vi "Check Upgrade.vi"(8 "error in (no error)":errorcluster, 11 "WebSocket Client in":refnum<class "WebSocket Client.lvclass">) -> (0 "error out":errorcluster, 1 "Is WS Upgrade":bool, 2 "Response":refnum<class "WebSocketUpgradeResponse.lvclass">, 3 "WebSocket Client out":refnum<class "WebSocket Client.lvclass">)   [LabVIEW 2020, in "HTTP Server.lvlib" / "WebSocket Client.lvclass"]
uses:
  WebSocket Client.lvclass
  WebSocket Client.lvclass/WebSocket Client.ctl
  lv-http-util/HTTP Utils/Request/Request.lvclass
  lv-http-util/HTTP Utils/Method.ctl
  lv-http-util/HTTP Utils/HTTP Utils.lvlib
  WebSocketUpgradeResponse/WebSocketUpgradeResponse.lvclass
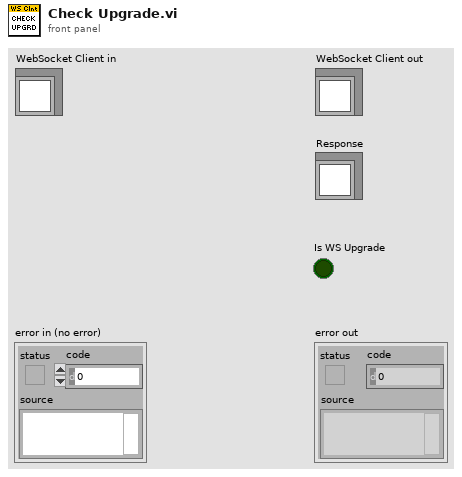
[diagram p1: front panel]
types:
  T1 = typedef "HTTP Utils.lvlib/Method.ctl" = enum16{"GET", "HEAD", "POST", "PUT", "DELETE", "CONNECT", "OPTIONS", "TRACE", "PATCH"}
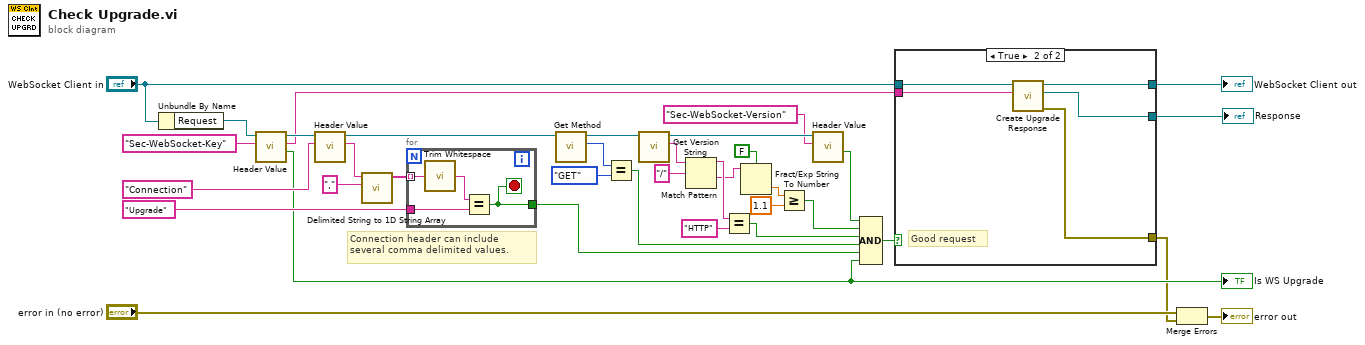
[diagram p0: block diagram]
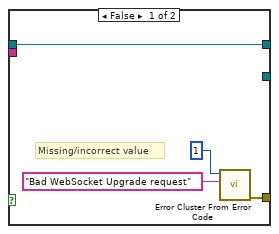
[diagram p2: hidden frame]
diagram:
  # "Connection header can include several comma delimited values."
  n1 = Unbundle By Name("WebSocket Client in") -> ("Request"=w8:refnum<class "Request.lvclass">)
  n2 = call "Header Value.vi"("Header"="Sec-WebSocket-Key", "Request in"=w8) -> ("Exists"=w7:bool, "Value"=w2:string, "Request out"=w34:refnum<class "Request.lvclass">)  [unwired: 6 in, 1 out]
  "Is WS Upgrade" <- w7
  n3 = call "Header Value.vi"("Header"="Connection", "Request in"=w34) -> ("Value"=w11:string, "Request out"=w30:refnum<class "Request.lvclass">)  [unwired: 6 in, 2 out]
  n4 = call <vilib>:"Delimited String to 1D String Array.vi"("delimiter"=",", "delimited string"=w11) -> ("string array"=w9:string[])  [unwired: 9 in]
  n5 = for {
    tunnel: "Upgrade" -> [w40]
    tunnel: [w37] -> w31
    tunnel: w9 -> [w39] mode=indexing
    stop <- w37 stop-if-true
    n6 = call <vilib>:"Trim Whitespace.vi"("string"=w39) -> ("trimmed string"=w38:string)  [unwired: 1 in]
    n7 = Equal?(x=w38, y=w40) -> (x = y?=w37:bool)
  }
  n8 = call "Get Method.vi"("Request in"=w30) -> ("Method"=w29:T1, "Request out"=w27:refnum<class "Request.lvclass">)  [unwired: 8 in, 1 out]
  n9 = Equal?(x=w29, y=Method."GET") -> (x = y?=w26:bool)
  n10 = call "Get Version String.vi"("Request in"=w27) -> ("Version String"=w25:string, "Request out"=w16:refnum<class "Request.lvclass">)  [unwired: 8 in, 1 out]
  n11 = Match Pattern(string=w25, regular expression="/") -> (before substring=w23:string, after substring=w21:string)  [unwired: 1 in, 2 out]
  n12 = Equal?(x=w23, y="HTTP") -> (x = y?=w19:bool)
  n13 = Fract/Exp String To Number(use system decimal point (T)=FALSE, string=w21) -> (number=w20:dbl)  [unwired: 2 in, 1 out]
  n14 = Greater Or Equal?(x=w20, y=1.1) -> (x >= y?=w17:bool)
  n15 = call "Header Value.vi"("Header"="Sec-WebSocket-Version", "Request in"=w16) -> ("Exists"=w14:bool)  [unwired: 6 in, 3 out]
  n16 = Compound Arithmetic op=AND(w14, w17, w19, w26, w31, w7) -> (w13:bool)
  n17 = case shown="True" w13 {
    tunnel: [w42 w47] -> w5
    tunnel: "WebSocket Client in" -> [w41 w49]
    tunnel: [w41 w46] -> w3
    tunnel: w2 -> [_ w48]
    tunnel: [_ w45] -> w1
    frame False {
      # "Missing/incorrect value"
      n18 = call <vilib>:"Error Cluster From Error Code.vi"("error message (\"\")"="Bad WebSocket Upgrade request" ("error message (\"\")"), "error code (0)"=1) -> ("error out"=w42:errorcluster)  [unwired: 7 in]
    }
    frame True {
      # "Good request"
      n19 = call "Create Upgrade Response.vi"("Sec-WebSocket-Key"=w48, "WebSocket Client in"=w49) -> ("error out"=w47:errorcluster, "WebSocketUpgradeResponse"=w45:refnum<class "WebSocketUpgradeResponse.lvclass">, "WebSocket Client out"=w46:refnum<class "WebSocket Client.lvclass">)  [unwired: 7 in]
    }
  }
  "WebSocket Client out" <- w3
  "Response" <- w1
  n20 = Merge Errors("error in (no error)", w5) -> (→"error out":errorcluster)
